vi "1.5.8-Insertion.vi"(6 "Opt: Timeout":u8=100, 7 "Counter Descriminator":u8, 8 "Input B":fxp<+/-,18,1>, 9 "Input A":fxp<+/-,18,1>, 10 "Channel Identifier":u8, 11 "FIFO":refnum<k21>="1.5.3-MultServ In") -> (0 "Timeout":bool)   [LabVIEW 2010]
doc: "Inserts a piece of data into a MultServer FIFO so it can be grabbed later"
uses:
  <vilib>/Platform/TimedLoop/XDataNode/XDataNode.xnode
  <vilib>/Platform/TimedLoop/XDataNode/timing_clust.ctl
  <vilib>/Platform/TimedLoop/XDataNode/nitl_modes.ctl
  <vilib>/Platform/TimedLoop/XDataNode/wakeup.ctl
  <vilib>/rvi/DataTransferAndStorage/Container/XNode/niFpgaContainer.xnode
  <vilib>/rvi/DataTransferAndStorage/Container/Common/niFpgaTransferTypeControl.ctl
  <vilib>/rvi/FIFO/Fifo_Types/niFpgaFifoControlLogicControl.ctl
  <vilib>/rvi/DataTransferAndStorage/Container/Common/niFpgaContainerMethod.ctl
  <vilib>/rvi/DataTransferAndStorage/Container/Common/niFpgaContainerMetaDataKey.ctl
  <vilib>/rvi/DataTransferAndStorage/FIFO/niFpgaPeerToPeerStreamState.ctl
  <vilib>/rvi/DataTransferAndStorage/Container/Common/niFpgaContainerExecOnDevCompGetState.vi
  <vilib>/rvi/FIFO/Fifo_Resource/nirvififoEmulationSetSize.vi
  <vilib>/rvi/DataTransferAndStorage/Container/Common/niFpgaContainerGetUniqueNameForEmu.vi
  <vilib>/rvi/interface/RandomDataEmulation/nirviRandomDataFPGAFIFO.vi
  <vilib>/rvi/interface/RandomDataEmulation/niFpgaRandomDataHandleErrors.vi
  <vilib>/rvi/eio/common/nirviEmuReportErrorAndStop.vi
  1.0-Hindbrain Global.vi
  <vilib>/Platform/TimedLoop/XDataNode/XDNodeRunTimeDep.lvlib
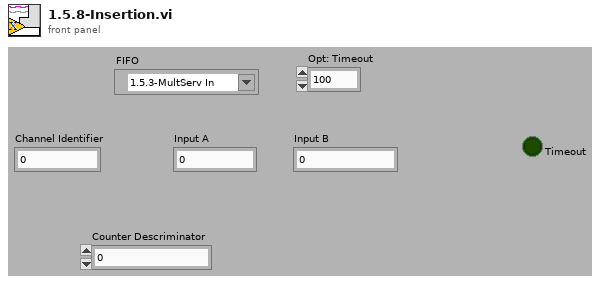
[diagram p1: front panel]
types:
  T1 = typedef "XDNodeRunTimeDep.lvlib/timing_clust.ctl" = cluster{"Expected End [f-1]":u64, "Actual End [f-1]":u64, "Finished Late? [f-1]":bool, "Expected End [i-1]":u64, "Actual End [i-1]":u64, "Finished Late? [i-1]":bool, "Expected Start [i]":u64, "Actual Start [i]":u64, "Expected Start [f]":u64, "Actual Start [f]":u64, "Source Name":string, "Structure Name":string, "Period":i64, "Deadline":i64, "Offset":i64, "Start":i64, "Priority":i32, "Timeout":i32, "Mode":T2, "Wakeup Reason":T3, "Error":errorcluster, "Source Type":string, "Secondary Source Type":string, "Global End Time":u64, "Global Start Time":u64, "Frame Duration":u64, "Iteration Duration":u64, "Assigned CPU":i32, "I/O Scan Engine Mode":u32}
  T2 = typedef "XDNodeRunTimeDep.lvlib/nitl_modes.ctl" = enum32{"No Change", "Process missed periods, maintain original phase", "Discard missed periods, maintain original phase", "Process missed periods, ignore original phase", "Discard missed periods, ignore original phase"}
  T3 = typedef "XDNodeRunTimeDep.lvlib/wakeup.ctl" = enum32{"Normal", "Aborted", "Asynchronous wakeup", "Timing source error", "Timed loop error", "Timeout"}
  T4 = typedef "niFpgaFifoControlLogicControl.ctl" = enum16{"Slice Fabric", "Target Optimal", "Built-in"}
  T5 = typedef "niFpgaContainerMethod.ctl" = enum16{"<none>", "write", "read", "clear", "getNumberOfElementsToWrite", "getNumberOfElementsToRead", "enable", "disable", "flushAndDisable", "getStreamState", "readA", "readB", "dramWrite", "dramWriteWithByteEnables", "dramRequestData", "dramRetrieveData"}
  T6 = typedef "niFpgaTransferTypeControl.ctl" = enum16{"Target-Scoped", "Host to Target - DMA", "Target to Host - DMA", "Peer to Peer Reader", "Peer to Peer Writer", "Bidirectional"}
  T7 = typedef "niFpgaPeerToPeerStreamState.ctl" = enum16{"Unlinked", "Disabled", "Enabled", "Flushing"}
  T8 = typedef "niFpgaContainerMetaDataKey.ctl" = enum16{"FPGA FIFO", "FPGA Memory", "FPGA Register"}
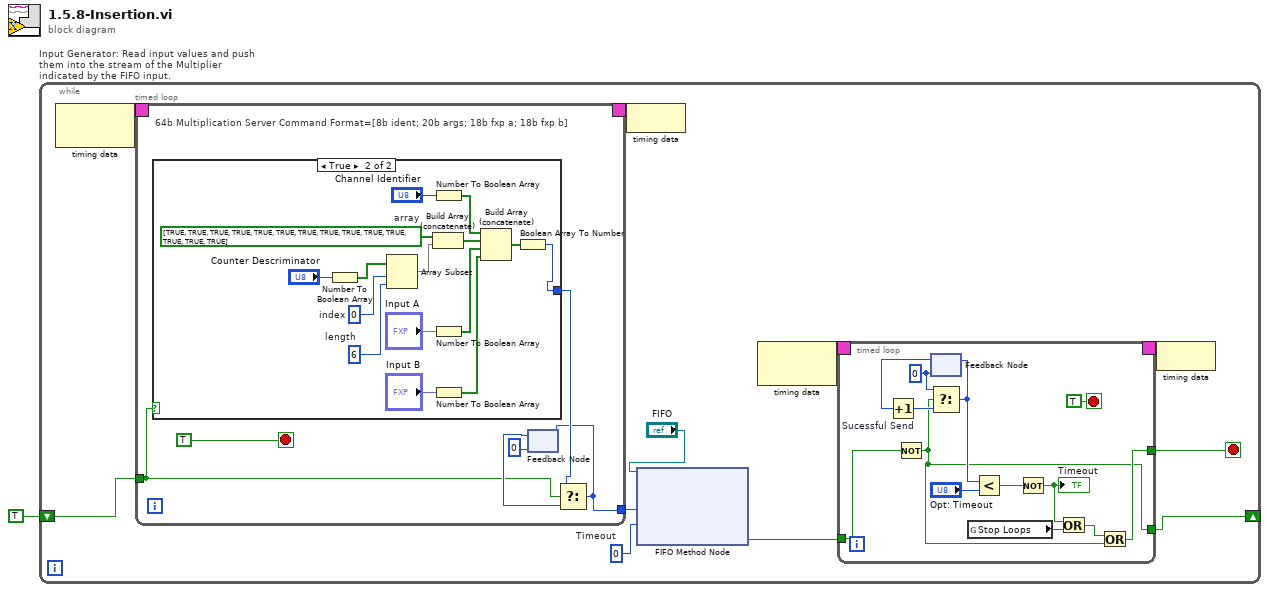
[diagram p0: block diagram]
diagram:
  n1 = while "Input Generator: Read input values and push them into the stream of the Multiplier indicated by the FIFO input." {
    shift-right: [w9] -> _
    shift-left: TRUE -> [w11]
    stop <- w10 stop-if-true
    w5 = 0  # Timeout
    n2 = node-c288() -> (w7:T1)  [unwired: 1 in]
    n3 = timed-loop {
      timing: w7 -> [_]
      timing-out: [_] -> w6
      tunnel: w11 -> [w33]
      tunnel: [w31] -> w8
      stop <- TRUE stop-if-true
      # "64b Multiplication Server Command Format=[8b ident; 20b args; 18b fxp a; 18b fxp b]"
      n4 = case shown="True" w33 {
        tunnel: [_ w46] -> w35
        frame False {
        }
        frame True {
          w39 = bool[] [TRUE, TRUE, TRUE, TRUE, TRUE, TRUE, TRUE, TRUE, TRUE, TRUE, TRUE, TRUE, TRUE, TRUE]  # array
          w40 = 6  # length
          w41 = 0  # index
          n5 = Number To Boolean Array(number="Counter Descriminator") -> (Boolean array=w42:bool[])
          n6 = Array Subset(array=w42, index=w41, length=w40) -> (w38:bool[])
          n7 = Build Array (concatenate)(w39, w38) -> (w37:bool[])
          n8 = Number To Boolean Array(number="Channel Identifier") -> (Boolean array=w49:bool[])
          n9 = Number To Boolean Array(number="Input A") -> (Boolean array=w48:bool[])
          n10 = Number To Boolean Array(number="Input B") -> (Boolean array=w47:bool[])
          n11 = Build Array (concatenate)(w49, w37, w48, w47) -> (w36:bool[])
          n12 = Boolean Array To Number(Boolean array=w36) -> (number=w46:u64)
        }
      }
      n13 = feedback #1(u64 0) -> (w34:u64)
      n14 = Select(t=w35, s=w33, f=w34) -> (s? t:f=w31:u64)
      n15 = feedback-in #1(w31) -> ()
    }
    n16 = node-c288(w6) -> ()
    n17 = xnode ("FIFO Method Node")("Element"=w8, "Timeout"=w5, "FIFO In"="FIFO") -> ("Timed Out?"=w12:bool)  [unwired: 1 out]
    n18 = node-c288() -> (w4:T1)  [unwired: 1 in]
    n19 = timed-loop {
      timing: w4 -> [_]
      timing-out: [_] -> w3
      tunnel: w12 -> [w25]
      tunnel: [w14] -> w10
      tunnel: [w13] -> w9
      stop <- TRUE stop-if-true
      w23 = u8 0
      n20 = Not "Sucessful Send"(x=w25) -> (.not. x?=w13:bool)
      n21 = feedback #2(w23) -> (w24:u8)
      n22 = Increment(x=w24) -> (x+1=w22:u8)
      n23 = Select(t=w23, s=w13, f=w22) -> (s? t:f=w21:u8)
      n24 = feedback-in #2(w21) -> ()
      n25 = global read "1.0-Hindbrain Global.vi" "Stop Loops"() -> (w15:bool)
      n26 = Less?(x=w21, y="Opt: Timeout") -> (x < y?=w19:bool)
      n27 = Not(x=w19) -> (.not. x?=w17:bool)
      "Timeout" <- w17
      n28 = Or(x=w17, y=w15) -> (x .or. y?=w18:bool)
      n29 = Or(x=w18, y=w13) -> (x .or. y?=w14:bool)
    }
    n30 = node-c288(w3) -> ()
  }
